vi "Opt2.vi"(0 "Activation Function":enum32{"Sigmoid", "RELU", "Tanh", "Leaky RELU"}(ring), 1 "Weights l+1":dbl[](array[numeric]), 2 "Weights":dbl[][](array[numeric]), 3 "Biases":dbl[](array[numeric]), 5 "Net Output":dbl[](array[numeric]), 7 "Activations l-1":dbl[](array[numeric]) format="%.2f", 9 "Delta l+1":dbl) -> (4 "Delta l":dbl[](array[numeric]), 13 "Updated Weights":dbl[][](array[numeric]), 14 "Updated Biases":dbl[](array[numeric]))   [LabVIEW 2018]
uses:
  <vilib>/Analysis/baseanly.llb/Real Outer Product.vi
  <vilib>/Analysis/Matrix/Numeric/Conversions/Matrix To Array - RM.vi
  Optimizer.vi
  Adam_data.vi
  Iteration Counter.vi
  <vilib>/Analysis/NI_AALBase.lvlib
  <vilib>/Analysis/Matrix/NI_Matrix.lvlib
panel:
  out "Grad. w":dbl[][](array[numeric])
  out "Grad. b":dbl[](array[numeric])
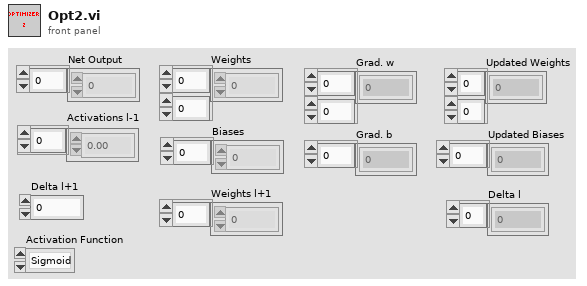
[diagram p1: front panel]
types:
  T1 = typedef "NI_Matrix.lvlib/RealMatrix.ctl" = dbl[][]
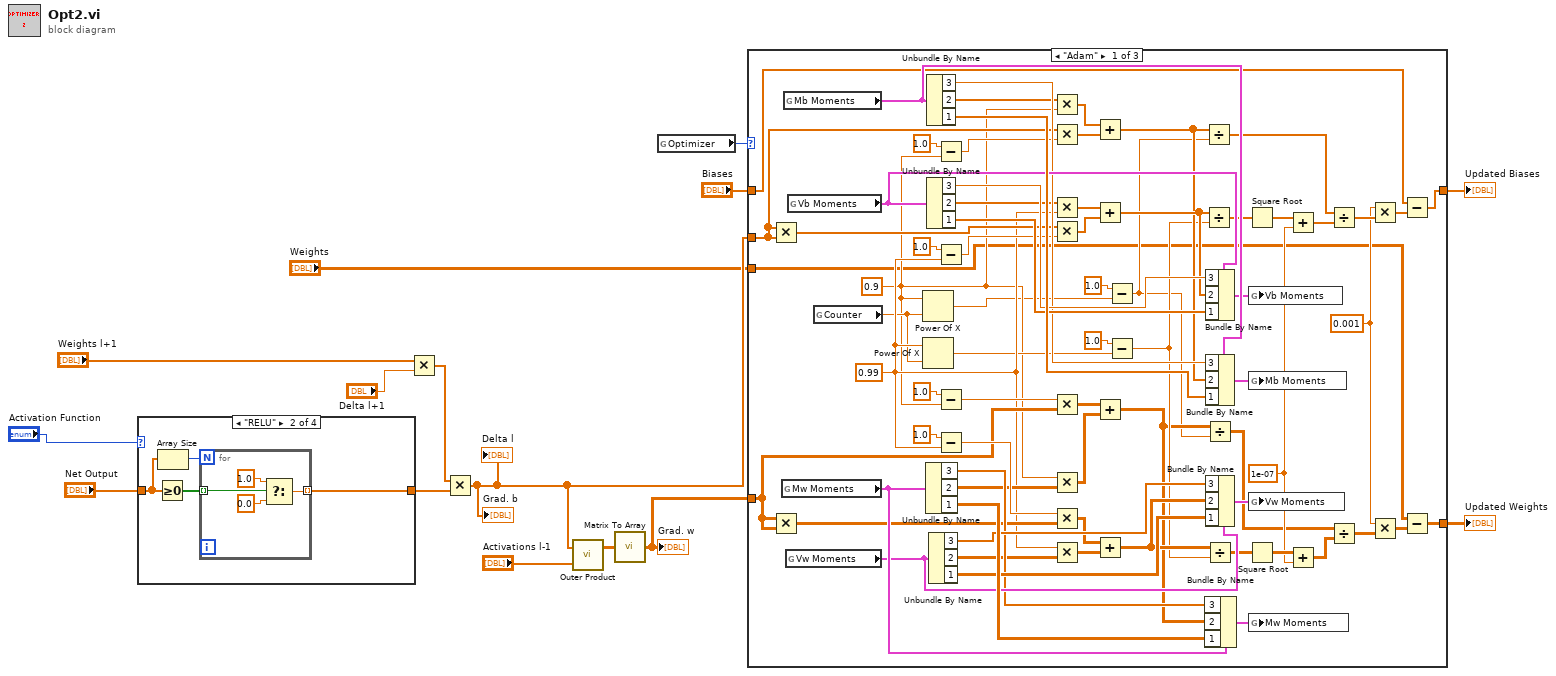
[diagram p0: block diagram]
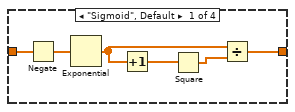
[diagram p4: hidden frame]
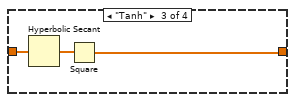
[diagram p5: hidden frame]
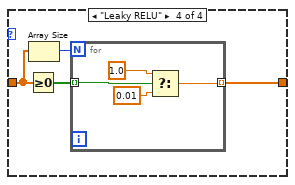
[diagram p6: hidden frame]
diagram:
  n1 = case shown="\"RELU\"" "Activation Function" {
    tunnel: "Net Output" -> [w17 w23 w31 w34]
    tunnel: [w16 w25 w30 w36] -> w14
    frame "Sigmoid", Default {
      n2 = Negate(x=w17) -> (-x=w21:dbl[])
      n3 = Exponential(1:w21) -> (0:w18:dbl[])
      n4 = Increment(x=w18) -> (x+1=w20:dbl[])
      n5 = Square(x=w20) -> (x^2=w19:dbl[])
      n6 = Divide(x=w18, y=w19) -> (x/y=w16:dbl[])
    }
    frame "RELU" {
      n7 = Greater Or Equal To 0?(x=w23) -> (x >= 0?=w24:bool[])
      n8 = Array Size(array=w23) -> (size(s)=w22:i32)
      n9 = for {
        N: w22 -> [_]
        tunnel: [w29] -> w25 mode=indexing
        tunnel: w24 -> [w26] mode=indexing
        n10 = Select(t=1.0, s=w26, f=0.0) -> (s? t:f=w29:dbl)
      }
    }
    frame "Tanh" {
      n11 = Hyperbolic Secant(1:w31) -> (0:w32:dbl[])
      n12 = Square(x=w32) -> (x^2=w30:dbl[])
    }
    frame "Leaky RELU" {
      n13 = Greater Or Equal To 0?(x=w34) -> (x >= 0?=w35:bool[])
      n14 = Array Size(array=w34) -> (size(s)=w33:i32)
      n15 = for {
        N: w33 -> [_]
        tunnel: [w38] -> w36 mode=indexing
        tunnel: w35 -> [w37] mode=indexing
        n16 = Select(t=1.0, s=w37, f=0.01) -> (s? t:f=w38:dbl)
      }
    }
  }
  n17 = Multiply(x="Weights l+1", y="Delta l+1") -> (x*y=w1:dbl[])
  n18 = Multiply(x=w1, y=w14) -> (x*y=w9:dbl[])
  "Grad. b" <- w9
  "Delta l" <- w9
  n19 = call-poly <vilib>:"Outer Product.vi"("Y Vector"="Activations l-1", "X Vector"=w9) -> ("Outer Product"=w8:T1)  [unwired: 1 out]
  n20 = call-poly <vilib>:"Matrix To Array.vi"("Real Matrix"=w8) -> ("Real 2D Array"=w7:dbl[][])
  "Grad. w" <- w7
  n21 = global read "Optimizer.vi" "Optimizer"() -> (w13:enum16{"Adagrad", "Adadelta", "Adam"})
  n22 = case shown="\"Adam\"" w13 {
    tunnel: "Weights" -> [w42 w113 w115]
    tunnel: [w41 w113 w115] -> w6
    tunnel: "Biases" -> [w45 w112 w114]
    tunnel: [w44 w112 w114] -> w11
    tunnel: w9 -> [w89 _ _]
    tunnel: w7 -> [w74 _ _]
    frame "Adam" {
      w51 = 1e-07
      w47 = 0.001
      w71 = 0.99
      w66 = 0.9
      n23 = Multiply(x=w89, y=w89) -> (x*y=w88:dbl[])
      n24 = Multiply(x=w74, y=w74) -> (x*y=w78:dbl[][])
      n25 = global read "Adam_data.vi" "Mw Moments"() -> (w110:cluster{"3 ":dbl[], "2":dbl[][], "1":dbl[][]})
      n26 = global read "Adam_data.vi" "Mb Moments"() -> (w105:cluster{"1":dbl[], "2":dbl[], "3":dbl})
      n27 = global read "Adam_data.vi" "Vw Moments"() -> (w108:cluster{"3":dbl[], "2":dbl[][], "1":dbl[][]})
      n28 = global read "Adam_data.vi" "Vb Moments"() -> (w102:cluster{"3":dbl, "2":dbl[], "1":dbl[]})
      n29 = global read "Iteration Counter.vi" "Counter"() -> (w67:dbl)
      n30 = Power Of X(1:w67, 2:w66) -> (0:w64:dbl)
      n31 = Power Of X(1:w67, 2:w71) -> (0:w70:dbl)
      n32 = Unbundle By Name(w110) -> ("3"=w84:dbl[], "2"=w77:dbl[][], "1"=w109:dbl[][])
      n33 = Unbundle By Name(w105) -> ("3"=w98:dbl, "2"=w97:dbl[], "1"=w104:dbl[])
      n34 = Unbundle By Name(w102) -> ("3"=w99:dbl, "2"=w92:dbl[], "1"=w101:dbl[])
      n35 = Unbundle By Name(w108) -> ("3"=w85:dbl[], "2"=w83:dbl[][], "1"=w107:dbl[][])
      n36 = Subtract(x=1.0, y=w66) -> (x-y=w95:dbl)
      n37 = Subtract(x=1.0, y=w71) -> (x-y=w90:dbl)
      n38 = Subtract(x=1.0, y=w66) -> (x-y=w75:dbl)
      n39 = Subtract(x=1.0, y=w71) -> (x-y=w81:dbl)
      n40 = Multiply(x=w97, y=w66) -> (x*y=w94:dbl[])
      n41 = Multiply(x=w89, y=w95) -> (x*y=w93:dbl[])
      n42 = Multiply(x=w92, y=w71) -> (x*y=w87:dbl[])
      n43 = Multiply(x=w88, y=w90) -> (x*y=w86:dbl[])
      n44 = Multiply(x=w75, y=w74) -> (x*y=w73:dbl[][])
      n45 = Multiply(x=w66, y=w77) -> (x*y=w72:dbl[][])
      n46 = Multiply ("Multiply.vi")(x=w81, y=w78) -> (x*y=w80:dbl[][])
      n47 = Multiply(x=w71, y=w83) -> (x*y=w79:dbl[][])
      n48 = Add(x=w94, y=w93) -> (x+y=w63:dbl[])
      n49 = Add(x=w87, y=w86) -> (x+y=w68:dbl[])
      n50 = Add(x=w73, y=w72) -> (x+y=w60:dbl[][])
      n51 = Add(x=w80, y=w79) -> (x+y=w62:dbl[][])
      n52 = Subtract(x=1.0, y=w64) -> (x-y=w59:dbl)
      n53 = Subtract(x=1.0, y=w70) -> (x-y=w61:dbl)
      n54 = Divide(x=w63, y=w59) -> (x/y=w55:dbl[])
      n55 = Divide(x=w68, y=w61) -> (x/y=w58:dbl[])
      n56 = Divide(x=w60, y=w59) -> (x/y=w50:dbl[][])
      n57 = Divide(x=w62, y=w61) -> (x/y=w53:dbl[][])
      n58 = Bundle By Name(cluster=w110, "3"=w84, "2"=w60, "1"=w109) -> (w111:cluster{"3 ":dbl[], "2":dbl[][], "1":dbl[][]})
      n59 = Bundle By Name(cluster=w102, "3"=w99, "2"=w68, "1"=w101) -> (w100:cluster{"3":dbl, "2":dbl[], "1":dbl[]})
      n60 = Bundle By Name(cluster=w105, "3"=w98, "2"=w63, "1"=w104) -> (w103:cluster{"1":dbl[], "2":dbl[], "3":dbl})
      n61 = Bundle By Name(cluster=w108, "3"=w85, "2"=w62, "1"=w107) -> (w106:cluster{"3":dbl[], "2":dbl[][], "1":dbl[][]})
      n62 = Square Root(x=w58) -> (sqrt(x)=w57:dbl[])
      n63 = Square Root(x=w53) -> (sqrt(x)=w52:dbl[][])
      n64 = global write "Adam_data.vi" "Vb Moments"(w100) -> ()
      n65 = global write "Adam_data.vi" "Mb Moments"(w103) -> ()
      n66 = global write "Adam_data.vi" "Vw Moments"(w106) -> ()
      n67 = global write "Adam_data.vi" "Mw Moments"(w111) -> ()
      n68 = Add(x=w57, y=w51) -> (x+y=w56:dbl[])
      n69 = Add(x=w52, y=w51) -> (x+y=w49:dbl[][])
      n70 = Divide(x=w55, y=w56) -> (x/y=w54:dbl[])
      n71 = Divide(x=w50, y=w49) -> (x/y=w48:dbl[][])
      n72 = Multiply(x=w47, y=w54) -> (x*y=w46:dbl[])
      n73 = Multiply(x=w47, y=w48) -> (x*y=w43:dbl[][])
      n74 = Subtract(x=w45, y=w46) -> (x-y=w44:dbl[])
      n75 = Subtract(x=w42, y=w43) -> (x-y=w41:dbl[][])
    }
    frame "Adadelta" {
    }
    frame "Adagrad" {
    }
  }
  "Updated Biases" <- w11
  "Updated Weights" <- w6
